vi "Enable Low-Band Filter.vi"(8 "error in (no error)":errorcluster, 10 "Enable Low-Band Filter (F: Disable)":bool, 11 "VISA resource name":refnum<visa-resource-name>) -> (0 "error out":errorcluster, 3 "VISA resource name out":refnum<visa-resource-name>)   [LabVIEW 2018, in "Agilent PSG MXG Series.lvlib"]
doc: "Enables or disables the low-band filter located in the RF path. This filter will reduce harmonics below 2 GHz.\n\n<B>Notes:</B>\n(1) This VI is valid only in PSG series."
uses:
  Agilent PSG MXG Series.lvlib
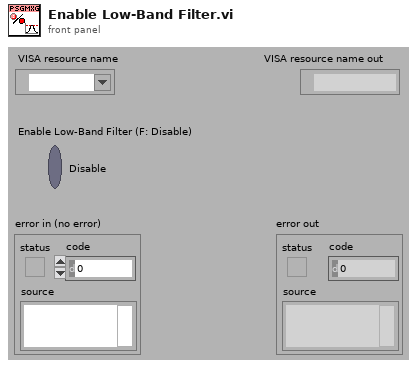
[diagram p1: front panel]
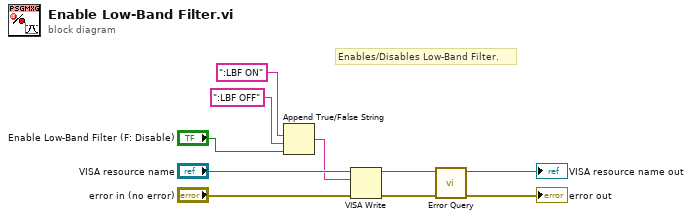
[diagram p0: block diagram]
diagram:
  # "Enables/Disables Low-Band Filter."
  n1 = Append True/False String(1:"Enable Low-Band Filter (F: Disable)", 2:":LBF OFF" ("write buffer"), 3:":LBF ON" ("write buffer")) -> (0:w2:string)  [unwired: 1 out]
  n2 = VISA Write(VISA resource name="VISA resource name", write buffer=w2, error in (no error)="error in (no error)") -> (VISA resource name out=w10:refnum<visa-resource-name>, error out=w9:errorcluster)  [unwired: 1 out]
  n3 = call "Error Query.vi"("error in (no error)"=w9, "VISA resource name"=w10) -> ("error out"=→"error out":errorcluster, "VISA resource name out"=→"VISA resource name out":refnum<visa-resource-name>)  [unwired: 8 out]
